vi "Initialize.vi"(8 "error in":errorcluster, 10 "parameters":variant, 11 "node in":refnum<class "AppStateMachine editor node.lvclass">) -> (0 "error out":errorcluster, 2 "summary":T2[](array[typedef]), 3 "data value reference":T1)   [LabVIEW 2017, in "AppStateMachine editor node.lvclass"]
doc: "Initializes the data of a node to its default state.\nThe object is not created inside of this VI, because it is created from a File depending on user selection."
uses:
  AppStateMachine editor node.lvclass
  C:/Program Files (x86)/National Instruments/LabVIEW 2017/vi.lib/NI/Configuration Framework/Node/NISE_CEF_Node.lvclass
  <vilib>/NI/Configuration Framework/Node/Summary.ctl
  <vilib>/NI/Configuration Framework/Node/NodeRef.ctl
  <vilib>/NI/Configuration Framework/Node/NISE_CEF_Node.lvclass
  module/configuration/AppStateMachine configuration.lvclass
  C:/Program Files (x86)/National Instruments/LabVIEW 2017/vi.lib/NI/Configuration Framework/serializable configuration/NISE_CEF_serializable configuration.lvclass
  module/configuration/AppStateMachine configuration.lvclass/AppStateMachine configuration.ctl
  module/configuration/Write PrechargeTimeout.vi
  module/configuration/Write SynchronizeTimeout.vi
  module/configuration/Write DCLinkSteadyStateTimeout.vi
  module/configuration/Write PrechargeLevel.vi
  module/configuration/Write DCLinkSteadyState.vi
  <vilib>/NI/DCAF/Tag Editor Core/control module/editor node/control module editor.lvclass
  <vilib>/NI/Configuration Framework/serializable configuration/NISE_CEF_serializable configuration.lvclass
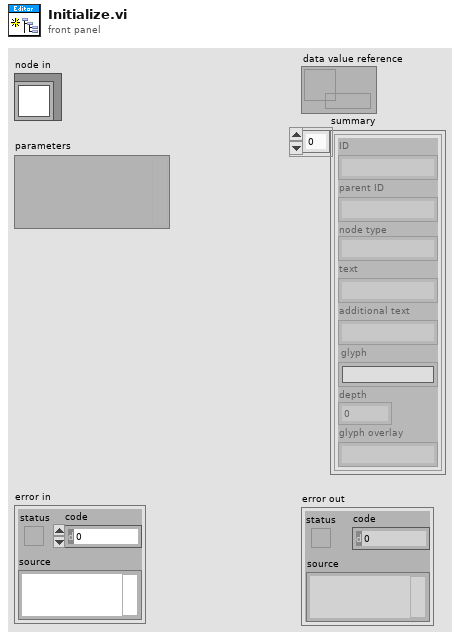
[diagram p1: front panel]
types:
  T1 = typedef "NISE_CEF_Node.lvclass/NodeRef.ctl" = refnum<data-value>
  T2 = typedef "NISE_CEF_Node.lvclass/Summary.ctl" = cluster{"ID":string, "parent ID":string, "node type":string, "text":string, "additional text":string, "glyph":string, "depth":i32, "glyph overlay":string}
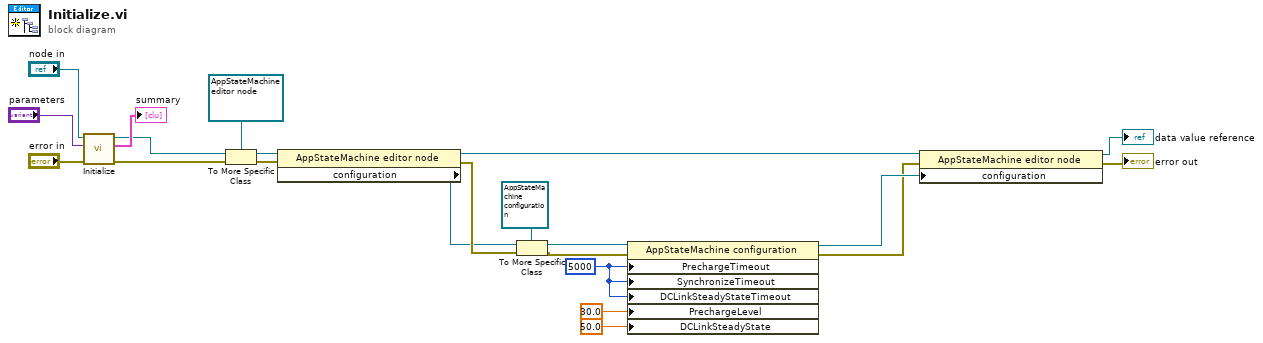
[diagram p0: block diagram]
diagram:
  w3 = u32 5000 ("PrechargeTimeout")
  n1 = call-parent "Initialize.vi"("error in"="error in", "parameters"="parameters", "node in"="node in") -> ("error out"=w9:errorcluster, "summary"=→"summary":T2[], "data value reference"=w10:T1)  [unwired: 6 in]
  n2 = To More Specific Class(target class=refnum<data-value> refnum ("data value reference"), reference=w10, error in=w9) -> (specific class reference=w18:refnum<data-value>, error out=w17:errorcluster)
  n3 = property class="AppStateMachine editor node"(reference=w18, error in=w17) -> (reference out=w14:refnum<data-value>, error out=w16:errorcluster, "configuration"=w15:refnum<class "NISE_CEF_serializable configuration.lvclass">)
  n4 = To More Specific Class(target class=refnum<class "AppStateMachine configuration.lvclass"> refnum ("AppStateMachine configuration"), reference=w15, error in=w16) -> (specific class reference=w5:refnum<class "AppStateMachine configuration.lvclass">, error out=w4:errorcluster)
  n5 = property class="AppStateMachine configuration"(reference=w5, error in=w4, "PrechargeTimeout"=w3, "SynchronizeTimeout"=w3, "DCLinkSteadyStateTimeout"=w3, "PrechargeLevel"=30.0, "DCLinkSteadyState"=50.0) -> (reference out=w13:refnum<class "AppStateMachine configuration.lvclass">, error out=w12:errorcluster)
  n6 = property class="AppStateMachine editor node"(reference=w14, error in=w12, "configuration"=w13) -> (reference out=→"data value reference":refnum<data-value>, error out=→"error out":errorcluster)
